vi "AutonomousVelocity.vi"() -> (0 "Terminate":bool)   [LabVIEW 2015]
uses:
  <vilib>/Rock Robotics/WPI/DriverStation/WPI_DriverStationRobotMode2.ctl
  <vilib>/Rock Robotics/WPI/CAN/TalonSRX/WPI_CANTalonSRX_APIControlMode.ctl
  <vilib>/Rock Robotics/WPI/Solenoid/WPI_SolenoidValue.ctl
  Utilities/AutoVars.vi
  Utilities/MotorPositionGlobals.vi
  Utilities/ShiftGlobals.vi
  Utilities/GlobalVisionVars.vi
  Utilities/VisionGlobals.vi
  <vilib>/Rock Robotics/WPI/Solenoid/WPI_SolenoidSetEnum.vi
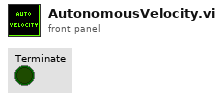
[diagram p1: front panel]
types:
  T1 = enum16{"WaitingForInput", "Driving", "TurnToTarget", "DriveMore", "Shoot", "End"}
  T2 = typedef "WPI_DriverStationRobotMode2.ctl" = enum16{"Autonomous Disabled", "Autonomous Enabled", "Teleop Disabled", "Teleop Enabled", "Disconnected", "Finish", "Test Disabled", "Test Enabled", "Emergency Stopped"}
  T3 = enum16{"Far Left", "Pos 2", "Pos 3", "Pos 4", "Far Right"}
  T4 = typedef "WPI_SolenoidValue.ctl" = enum16{"Off", "On", "Forward", "Reverse"}
  T5 = typedef "WPI_MotorControlDeviceRef.ctl" = cluster{"DeviceStatus":errorcluster, "Type":T6, "PWM":cluster{"PWM Channel":T7, "DeadBand":T8}, "CAN":cluster{"Device Number":u8, "Control Mode":T9, "Semaphore":T10, "Max Vout":dbl, "TalonSRX Control Mode":T11}, "Invert":bool}
  T6 = typedef "WPI_MotorControlType.ctl" = enum16{"PWM", "CAN", "CANTalonSRX"}
  T7 = typedef "FPGA_DIOPWMChannel.ctl" = enum8{"PWM 0", "PWM 1", "PWM 2", "PWM 3", "PWM 4", "PWM 5", "PWM 6", "PWM 7", "PWM 8", "PWM 9", "PWM MXP 0", "PWM MXP 1", "PWM MXP 2", "PWM MXP 3", "PWM MXP 4", "PWM MXP 5", "PWM MXP 6", "PWM MXP 7", "PWM MXP 8", "PWM MXP 9", "Invalid"}
  T8 = typedef "WPI_PWMDeadband.ctl" = cluster{"Name":string, "maxPositivePwm":i32, "minPositivePwm":i32, "centerPwm":i32, "maxNegativePwm":i32, "minNegativePwm":i32, "angularRange":u16}
  T9 = typedef "WPI_CANJaguar_ControlMode.ctl" = enum8{"Percent VBus", "Current", "Speed", "Position", "Voltage"}
  T10 = typedef "Semaphore RefNum" = refnum<k1>
  T11 = typedef "WPI_CANTalonSRX_APIControlMode.ctl" = enum8{"Percent VBus", "Speed", "Position", "Slave", "Unchanged / Invalid", "Voltage Compensation", "Current", "Motion Profile"}
  T12 = typedef "WPI_CANTalonSRX_GlobalStatus.ctl" = cluster{"Applied Throttle":dbl, "Module Enabled":bool, "CAN Error":errorcluster, "Closed Loop Error":dbl, "Forward Limit Switch Closed":bool, "Reverse Limit Switch Closed":bool, "Sensor Position":dbl, "Sensor Velocity":dbl, "Current":dbl, "Sticky Fault - Over Temp":bool, "Sticky Fault - Under Voltage":bool, "Sticky Fault - Forward Limit":bool, "Sticky Fault - Reverse Limit":bool, "Sticky Fault - Forward Soft Limit":bool, "Sticky Fault - Reverse Soft Limit":bool, "Brake is Enabled":bool, "Encoder Position":dbl, "Encoder Velocity":dbl, "Encoder Index Count":dbl, "Encoder A Pin State":bool, "Encoder B Pin State":bool, "Encoder Index Pin State":bool, "Analog In":dbl, "Analog In Velocity":dbl, "Temperature (C)":dbl, "Battery Voltage":dbl, "Control 5 Is Supported":bool, "Current Profile Slot Select":dbl, "Pos Div 8":bool, "Vel Div 4":bool, "Pulse Width Position":i32, "Pulse Width Velocity":i32, "Pulse Width Rise To Rise (us)":i32, "Pulse Width Rise To Fall (us)":i32, "Mot Prof Active Is Under Run":bool, "Mot Prof Active Has Under Run":bool, "Mot Prof Active Is Last":bool, "Mot Prof Active Velocity Only":bool, "Mot Prof Active Is Valid":bool, "Mot Prof Buffer Is Full":bool, "Mot Prof Active Profile Slot Select":i32, "Mot Prof NextID":i32, "Mot Prof Count":i32, "Mot Prof Active Velocity":dbl, "Mot Prof Active Position":dbl, "Mot Prof Output Enable":i32}
  T13 = typedef "WPI_DigitalOutputDevRef.ctl" = cluster{"DIO Channel":T14, "DevStatus":errorcluster}
  T14 = typedef "FPGA_DIOChannel.ctl" = enum8{"DIO 0", "DIO 1", "DIO 2", "DIO 3", "DIO 4", "DIO 5", "DIO 6", "DIO 7", "DIO 8", "DIO 9", "DIO MXP 0", "DIO MXP 1", "DIO MXP 2", "DIO MXP 3", "DIO MXP 4", "DIO MXP 5", "DIO MXP 6", "DIO MXP 7", "DIO MXP 8", "DIO MXP 9", "DIO MXP 10", "DIO MXP 11", "DIO MXP 12", "DIO MXP 13", "DIO MXP 14", "DIO MXP 15", "Invalid"}
  T15 = typedef "WPI_GyroDevRef.ctl" = cluster{"DevStatus":errorcluster, "Analog Channel":T16, "Offset":dbl, "Gain (VoltsPerDegree/Second)":dbl, "Gyro Type":enum16{"Analog", "XRS450"}, "Handle":i32, "SPI Bus":T17, "Device Found":bool, "Sample Rate":dbl, "Calibrate On Open":bool}
  T16 = typedef "FPGA_AIChannel.ctl" = enum8{"AI 0", "AI 1", "AI 2", "AI 3", "AI MXP 0", "AI MXP 1", "AI MXP 2", "AI MXP 3", "Invalid"}
  T17 = typedef "spi_bus.ctl" = enum16{"SPI On-Board, CS0", "SPI On-Board, CS1", "SPI On-Board, CS2", "SPI On-Board, CS3", "SPI MXP", "Invalid"}
  T18 = typedef "WPI_SolenoidDevRef.ctl" = cluster{"DevStatus":errorcluster, "Pneumatics Control Module":u8, "Forward Solenoid Channel":T19, "Reverse Solenoid Channel":T19}
  T19 = typedef "WPI_SolenoidChannel.ctl" = enum8{"Solenoid 0", "Solenoid 1", "Solenoid 2", "Solenoid 3", "Solenoid 4", "Solenoid 5", "Solenoid 6", "Solenoid 7", "Invalid"}
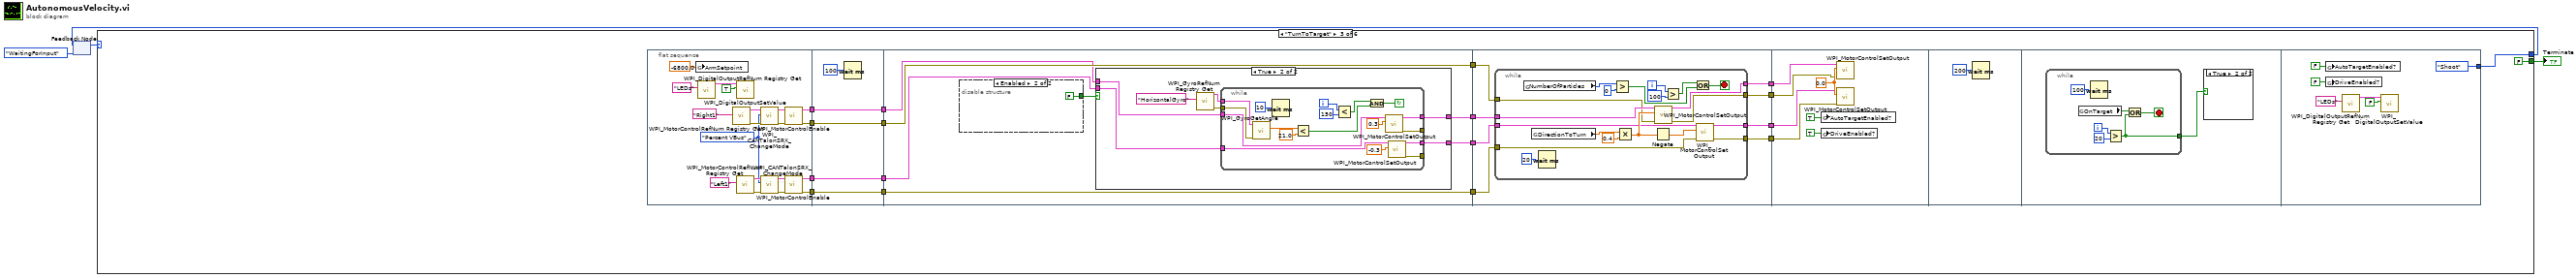
[diagram p0: block diagram]
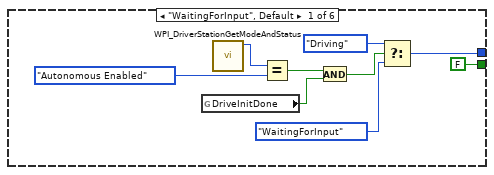
[diagram p2: hidden frame]
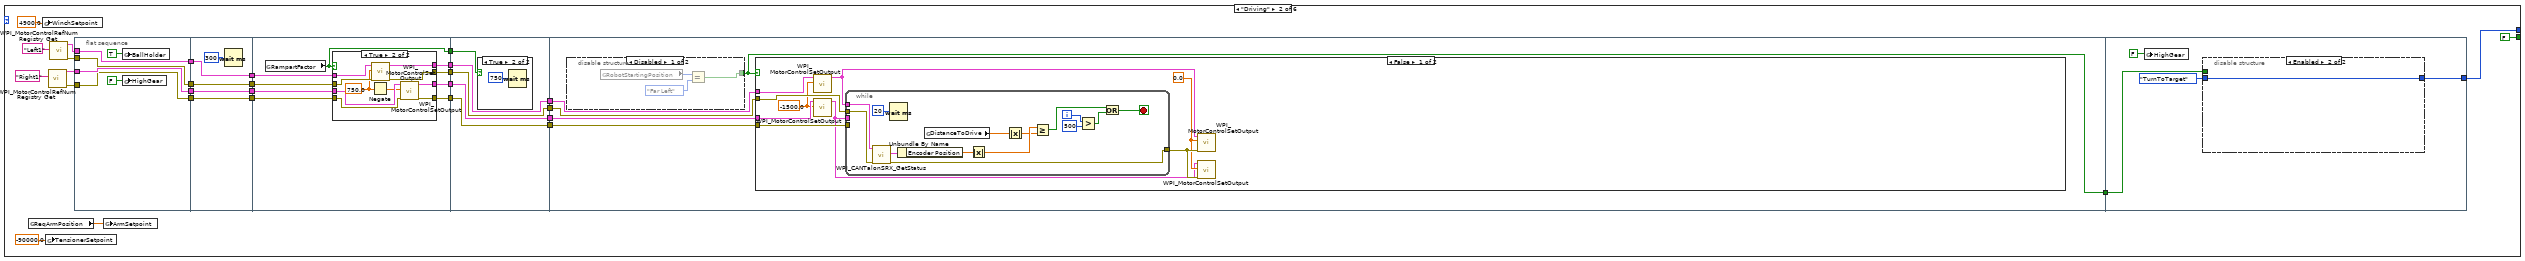
[diagram p3: hidden frame]
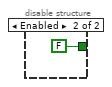
[diagram p6: hidden frame]
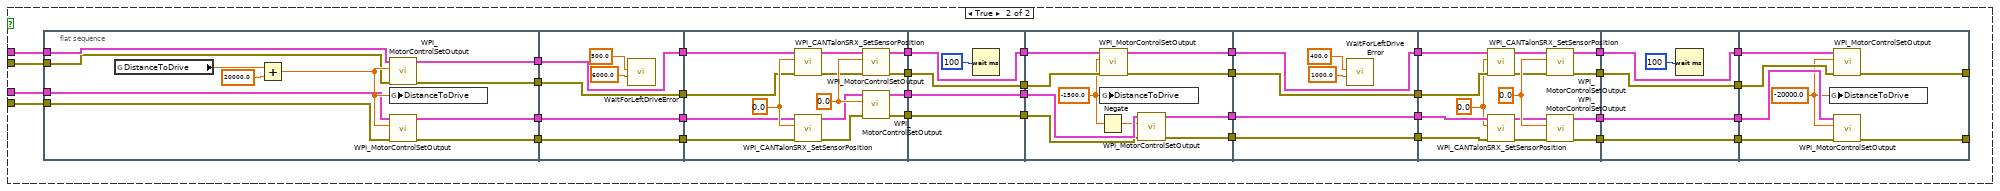
[diagram p7: hidden frame]
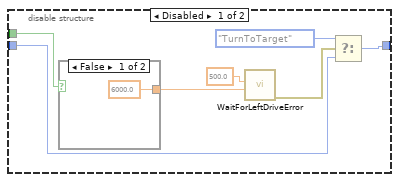
[diagram p8: hidden frame]
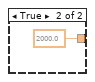
[diagram p9: hidden frame]
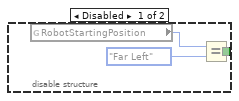
[diagram p10: hidden frame]
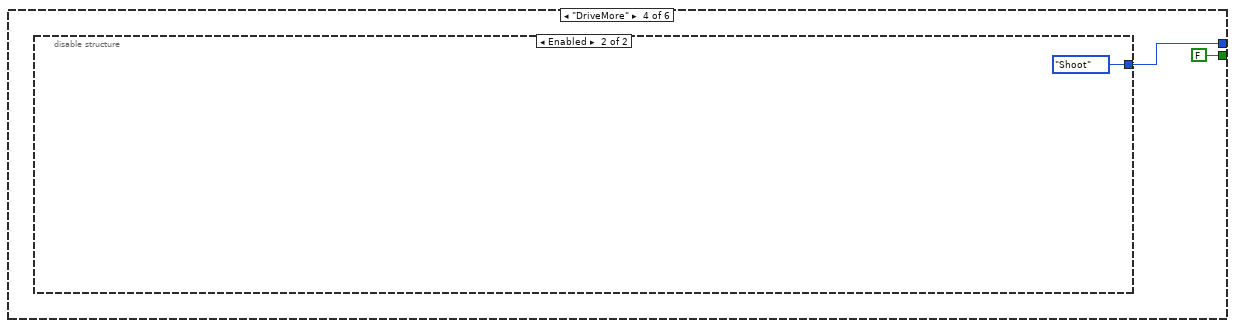
[diagram p13: hidden frame]
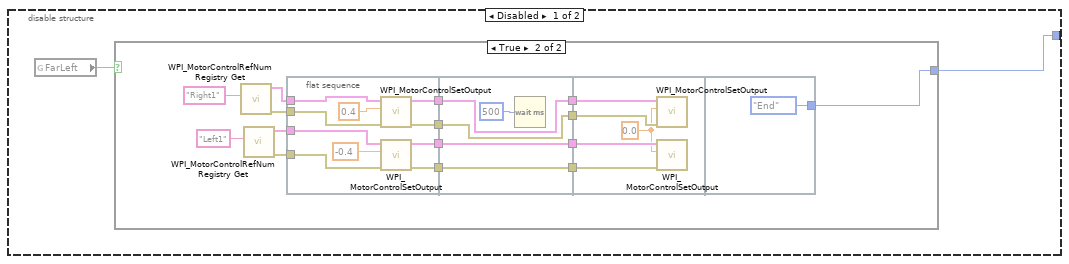
[diagram p14: hidden frame]
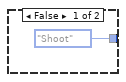
[diagram p15: hidden frame]
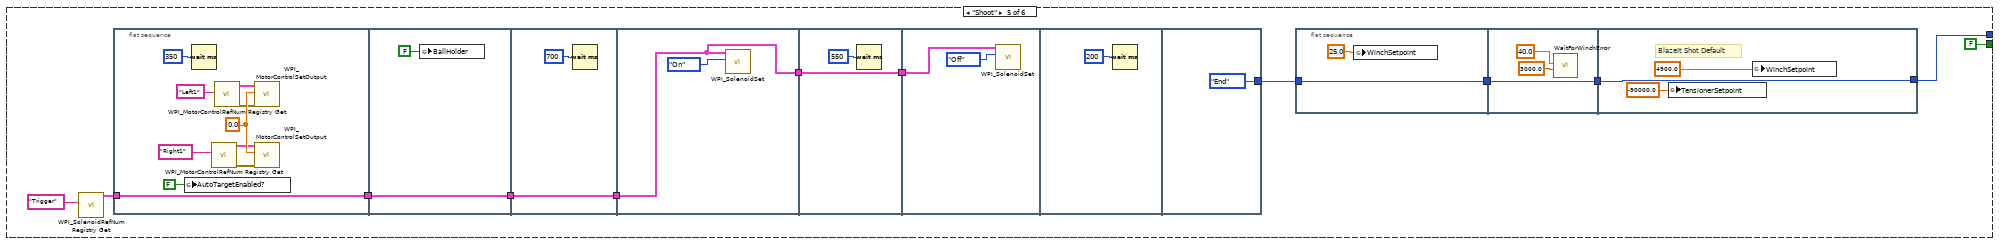
[diagram p16: hidden frame]
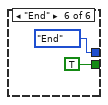
[diagram p17: hidden frame]
diagram:
  n1 = feedback #1(T1."WaitingForInput" ("AutoStateMachine")) -> (w1:T1)
  n2 = case shown="\"TurnToTarget\"" w1 {
    tunnel: [w13 w25 w260 w373 w416 T1."End" ("AutoStateMachine")] -> w4
    tunnel: [FALSE FALSE FALSE FALSE FALSE TRUE] -> w3
    frame "WaitingForInput", Default {
      n3 = global read "AutoVars.vi" "DriveInitDone"() -> (w8:bool)
      n4 = call <vilib>:"WPI_DriverStationGetModeAndStatus.vi"() -> ("Robot Mode"=w11:T2)  [unwired: 10 in, 1 out]
      n5 = Equal?(x=w11, y=WPI_DriverStationRobotMode2."Autonomous Enabled" ("Robot Mode")) -> (x = y?=w9:bool)
      n6 = And(x=w9, y=w8) -> (x .and. y?=w7:bool)
      n7 = Select(t=T1."Driving" ("AutoStateMachine"), s=w7, f=T1."WaitingForInput" ("AutoStateMachine")) -> (s? t:f=w13:T1)
    }
    frame "Driving" {
      n8 = global read "AutoVars.vi" "ReqArmPosition"() -> (w24:dbl)
      n9 = global write "MotorPositionGlobals.vi" "WinchSetpoint"(4900.0 ("WinchSetpoint")) -> ()
      n10 = global write "MotorPositionGlobals.vi" "TensionerSetpoint"(-90000.0 ("TensionerSetpoint")) -> ()
      n11 = call <vilib>:"WPI_MotorControlRefNum Registry Get.vi"("refnum name"="Right1") -> ("error out"=w36:errorcluster, "MotorControlDevRef"=w37:T5)  [unwired: 9 in]
      n12 = call <vilib>:"WPI_MotorControlRefNum Registry Get.vi"("refnum name"="Left1") -> ("error out"=w34:errorcluster, "MotorControlDevRef"=w35:T5)  [unwired: 9 in]
      n13 = flat-sequence {
        tunnel: w34 -> [w45]
        tunnel: w35 -> [w46]
        tunnel: w36 -> [w47]
        tunnel: w37 -> [w48]
        tunnel: [w48] -> w23
        tunnel: [w47] -> w21
        tunnel: [w46] -> w19
        tunnel: [w45] -> w17
        tunnel: w23 -> [w53]
        tunnel: [w53] -> w22
        tunnel: w21 -> [w52]
        tunnel: [w52] -> w20
        tunnel: w19 -> [w51]
        tunnel: [w51] -> w18
        tunnel: w17 -> [w50]
        tunnel: [w50] -> w16
        tunnel: [w58] -> w33
        tunnel: [w57] -> w31
        tunnel: [w56] -> w29
        tunnel: [w55] -> w27
        tunnel: w22 -> [w62]
        tunnel: w20 -> [w61]
        tunnel: w18 -> [w60]
        tunnel: w16 -> [w59]
        tunnel: [w54] -> w15
        tunnel: w33 -> [w81]
        tunnel: [w81] -> w32
        tunnel: w31 -> [w80]
        tunnel: [w80] -> w30
        tunnel: w29 -> [w79]
        tunnel: [w79] -> w28
        tunnel: w27 -> [w78]
        tunnel: [w78] -> w26
        tunnel: w15 -> [w77]
        tunnel: w32 -> [w87]
        tunnel: w30 -> [w86]
        tunnel: w28 -> [w84]
        tunnel: w26 -> [w85]
        tunnel: [w83] -> w14
        tunnel: [w231] -> w25
        tunnel: w14 -> [w230]
        frame #0 {
          n14 = global write "MotorPositionGlobals.vi" "BallHolder"(TRUE ("BallHolder")) -> ()
          n15 = global write "ShiftGlobals.vi" "HighGear"(FALSE ("HighGear")) -> ()
        }
        frame #1 {
          n16 = Wait (ms)(milliseconds to wait=u32 300) -> ()  [unwired: 1 out]
        }
        frame #2 {
          n17 = global read "AutoVars.vi" "RampartFactor"() -> (w54:bool)
          n18 = case shown="True" w54 {
            tunnel: w62 -> [w64 w76]
            tunnel: w61 -> [w63 w75]
            tunnel: w60 -> [w66 w74]
            tunnel: w59 -> [w65 w73]
            tunnel: [w64 w72] -> w58
            tunnel: [w63 w71] -> w57
            tunnel: [w66 w70] -> w56
            tunnel: [w65 w69] -> w55
            frame False {
            }
            frame True {
              w68 = 750.0
              n19 = Negate(x=w68) -> (-x=w67:dbl)
              n20 = call <vilib>:"WPI_MotorControlSetOutput.vi"("error in (no error)"=w73, "Output"=w68, "MotorControlDevRef"=w74) -> ("error out"=w69:errorcluster, "MotorControlDevRef"=w70:T5)  [unwired: 6 in, 1 out]
              n21 = call <vilib>:"WPI_MotorControlSetOutput.vi"("error in (no error)"=w75, "Output"=w67, "MotorControlDevRef"=w76) -> ("error out"=w71:errorcluster, "MotorControlDevRef"=w72:T5)  [unwired: 6 in, 1 out]
            }
          }
        }
        frame #3 {
          n22 = case shown="True" w77 {
            frame False {
            }
            frame True {
              n23 = Wait (ms)(milliseconds to wait=u32 750) -> ()  [unwired: 1 out]
            }
          }
        }
        frame #4 {
          n24 = disable-structure shown="Disabled" {
            disable-tunnel: [w88 FALSE] -> w83
            frame Disabled {
              n25 = global read "AutoVars.vi" "RobotStartingPosition"() -> (w90:T3)
              n26 = Equal?(x=w90, y=T3."Far Left") -> (x = y?=w88:bool)
            }
            frame Enabled {
            }
          }
          n27 = case shown="False" w83 {
            tunnel: w87 -> [w94 w149]
            tunnel: w86 -> [w99 w147]
            tunnel: w85 -> [w100 w148]
            tunnel: w84 -> [w96 w150]
            frame False {
              w92 = -1500.0 ("Output")
              w97 = 0.0 ("Output")
              n28 = call <vilib>:"WPI_MotorControlSetOutput.vi"("Output"=w92, "MotorControlDevRef"=w96) -> ("MotorControlDevRef"=w95:T5)  [unwired: 7 in, 2 out]
              n29 = call <vilib>:"WPI_MotorControlSetOutput.vi"("Output"=w92, "MotorControlDevRef"=w94) -> ("MotorControlDevRef"=w93:T5)  [unwired: 7 in, 2 out]
              n30 = while {
                tunnel: w93 -> [_]
                tunnel: w95 -> [w102]
                tunnel: w100 -> [w101]
                tunnel: w99 -> [_]
                tunnel: [w111] -> w98
                i -> [w107]
                stop <- w109 stop-if-true
                n31 = call <vilib>:"WPI_CANTalonSRX_GetStatus.vi"("error in (no error)"=w101, "CAN Talon SRX Ref"=w102) -> ("error out"=w111:errorcluster, "Talon SRX Status"=w113:T12)  [unwired: 7 in, 1 out]
                n32 = Wait (ms)(milliseconds to wait=u32 20) -> ()  [unwired: 1 out]
                n33 = Unbundle By Name(w113) -> ("Encoder Position"=w105:dbl)
                n34 = global read "AutoVars.vi" "DistanceToDrive"() -> (w112:dbl)
                n35 = Absolute Value(x=w105) -> (abs(x)=w104:dbl)
                n36 = Absolute Value(x=w112) -> (abs(x)=w103:dbl)
                n37 = Greater Or Equal?(x=w104, y=w103) -> (x >= y?=w110:bool)
                n38 = Greater?(x=w107, y=500) -> (0:w108:bool)
                n39 = Or(x=w110, y=w108) -> (x .or. y?=w109:bool)
              }
              n40 = call <vilib>:"WPI_MotorControlSetOutput.vi"("error in (no error)"=w98, "Output"=w97, "MotorControlDevRef"=w95) -> ()  [unwired: 6 in, 3 out]
              n41 = call <vilib>:"WPI_MotorControlSetOutput.vi"("error in (no error)"=w98, "Output"=w97, "MotorControlDevRef"=w93) -> ()  [unwired: 6 in, 3 out]
            }
            frame True {
              n42 = flat-sequence {
                tunnel: w150 -> [w158]
                tunnel: w149 -> [w157]
                tunnel: w148 -> [w156]
                tunnel: w147 -> [w155]
                tunnel: [w154] -> w145
                tunnel: [w153] -> w143
                tunnel: [w152] -> w141
                tunnel: [w151] -> w140
                tunnel: [w165] -> w146
                tunnel: w145 -> [w165]
                tunnel: [w164] -> w144
                tunnel: w143 -> [w164]
                tunnel: [w163] -> w142
                tunnel: w141 -> [w163]
                tunnel: w140 -> [w162]
                tunnel: [w162] -> w139
                tunnel: w146 -> [w175]
                tunnel: w144 -> [w174]
                tunnel: w142 -> [w173]
                tunnel: w139 -> [w172]
                tunnel: [w171] -> w130
                tunnel: [w170] -> w128
                tunnel: [w169] -> w126
                tunnel: [w168] -> w124
                tunnel: w130 -> [w186]
                tunnel: [w186] -> w129
                tunnel: w128 -> [w185]
                tunnel: [w185] -> w127
                tunnel: w126 -> [w184]
                tunnel: [w184] -> w125
                tunnel: w124 -> [w183]
                tunnel: [w183] -> w123
                tunnel: w129 -> [w196]
                tunnel: w127 -> [w195]
                tunnel: w125 -> [w194]
                tunnel: w123 -> [w193]
                tunnel: [w192] -> w138
                tunnel: [w191] -> w136
                tunnel: [w190] -> w134
                tunnel: [w189] -> w132
                tunnel: w138 -> [w202]
                tunnel: [w202] -> w137
                tunnel: w136 -> [w201]
                tunnel: [w201] -> w135
                tunnel: w134 -> [w200]
                tunnel: [w200] -> w133
                tunnel: w132 -> [w199]
                tunnel: [w199] -> w131
                tunnel: w137 -> [w215]
                tunnel: w135 -> [w214]
                tunnel: w133 -> [w213]
                tunnel: w131 -> [w212]
                tunnel: [w210] -> w116
                tunnel: [w209] -> w118
                tunnel: [w208] -> w120
                tunnel: [w207] -> w122
                tunnel: w122 -> [w221]
                tunnel: [w221] -> w121
                tunnel: w120 -> [w220]
                tunnel: [w220] -> w119
                tunnel: w118 -> [w219]
                tunnel: [w219] -> w117
                tunnel: w116 -> [w218]
                tunnel: [w218] -> w115
                tunnel: w121 -> [w225]
                tunnel: w119 -> [w226]
                tunnel: w117 -> [w227]
                tunnel: w115 -> [w228]
                tunnel: [w224] -> _
                tunnel: [w223] -> _
                frame #0 {
                  n43 = global read "AutoVars.vi" "DistanceToDrive"() -> (w160:dbl)
                  n44 = Add(x=w160, y=20000.0) -> (x+y=w159:dbl)
                  n45 = call <vilib>:"WPI_MotorControlSetOutput.vi"("error in (no error)"=w156, "Output"=w159, "MotorControlDevRef"=w158) -> ("error out"=w153:errorcluster, "MotorControlDevRef"=w154:T5)  [unwired: 6 in, 1 out]
                  n46 = global write "AutoVars.vi" "DistanceToDrive"(w159) -> ()
                  n47 = call <vilib>:"WPI_MotorControlSetOutput.vi"("error in (no error)"=w155, "Output"=w159, "MotorControlDevRef"=w157) -> ("error out"=w151:errorcluster, "MotorControlDevRef"=w152:T5)  [unwired: 6 in, 1 out]
                }
                frame #1 {
                  n48 = call "WaitForLeftDriveError.vi"("Timeout (ms)"=6000.0, "AllowedError"=500.0) -> ()  [unwired: 9 in, 1 out]
                }
                frame #2 {
                  w180 = 0.0 ("New Sensor Position")
                  w181 = 0.0 ("Output")
                  n49 = call <vilib>:"WPI_CANTalonSRX_SetSensorPosition.vi"("error in (no error)"=w174, "New Sensor Position"=w180, "CAN Talon SRX Ref"=w175) -> ("error out"=w178:errorcluster, "CAN Talon SRX Ref"=w179:T5)  [unwired: 7 in]
                  n50 = call <vilib>:"WPI_CANTalonSRX_SetSensorPosition.vi"("error in (no error)"=w172, "New Sensor Position"=w180, "CAN Talon SRX Ref"=w173) -> ("error out"=w176:errorcluster, "CAN Talon SRX Ref"=w177:T5)  [unwired: 7 in]
                  n51 = call <vilib>:"WPI_MotorControlSetOutput.vi"("error in (no error)"=w178, "Output"=w181, "MotorControlDevRef"=w179) -> ("error out"=w170:errorcluster, "MotorControlDevRef"=w171:T5)  [unwired: 6 in, 1 out]
                  n52 = call <vilib>:"WPI_MotorControlSetOutput.vi"("error in (no error)"=w176, "Output"=w181, "MotorControlDevRef"=w177) -> ("error out"=w168:errorcluster, "MotorControlDevRef"=w169:T5)  [unwired: 6 in, 1 out]
                }
                frame #3 {
                  n53 = Wait (ms)(milliseconds to wait=u32 100) -> ()  [unwired: 1 out]
                }
                frame #4 {
                  w187 = -1500.0
                  n54 = Negate(x=w187) -> (-x=w188:dbl)
                  n55 = call <vilib>:"WPI_MotorControlSetOutput.vi"("error in (no error)"=w195, "Output"=w187, "MotorControlDevRef"=w196) -> ("error out"=w191:errorcluster, "MotorControlDevRef"=w192:T5)  [unwired: 6 in, 1 out]
                  n56 = global write "AutoVars.vi" "DistanceToDrive"(w187) -> ()
                  n57 = call <vilib>:"WPI_MotorControlSetOutput.vi"("error in (no error)"=w193, "Output"=w188, "MotorControlDevRef"=w194) -> ("error out"=w189:errorcluster, "MotorControlDevRef"=w190:T5)  [unwired: 6 in, 1 out]
                }
                frame #5 {
                  n58 = call "WaitForLeftDriveError.vi"("Timeout (ms)"=1000.0, "AllowedError"=400.0) -> ()  [unwired: 9 in, 1 out]
                }
                frame #6 {
                  w211 = 0.0 ("New Sensor Position")
                  w216 = 0.0 ("Output")
                  n59 = call <vilib>:"WPI_CANTalonSRX_SetSensorPosition.vi"("error in (no error)"=w214, "New Sensor Position"=w211, "CAN Talon SRX Ref"=w215) -> ("error out"=w205:errorcluster, "CAN Talon SRX Ref"=w206:T5)  [unwired: 7 in]
                  n60 = call <vilib>:"WPI_CANTalonSRX_SetSensorPosition.vi"("error in (no error)"=w212, "New Sensor Position"=w211, "CAN Talon SRX Ref"=w213) -> ("error out"=w203:errorcluster, "CAN Talon SRX Ref"=w204:T5)  [unwired: 7 in]
                  n61 = call <vilib>:"WPI_MotorControlSetOutput.vi"("error in (no error)"=w205, "Output"=w216, "MotorControlDevRef"=w206) -> ("error out"=w209:errorcluster, "MotorControlDevRef"=w210:T5)  [unwired: 6 in, 1 out]
                  n62 = call <vilib>:"WPI_MotorControlSetOutput.vi"("error in (no error)"=w203, "Output"=w216, "MotorControlDevRef"=w204) -> ("error out"=w207:errorcluster, "MotorControlDevRef"=w208:T5)  [unwired: 6 in, 1 out]
                }
                frame #7 {
                  n63 = Wait (ms)(milliseconds to wait=u32 100) -> ()  [unwired: 1 out]
                }
                frame #8 {
                  w222 = -20000.0 ("Output")
                  n64 = global write "AutoVars.vi" "DistanceToDrive"(w222) -> ()
                  n65 = call <vilib>:"WPI_MotorControlSetOutput.vi"("error in (no error)"=w227, "Output"=w222, "MotorControlDevRef"=w228) -> ("error out"=w224:errorcluster)  [unwired: 6 in, 2 out]
                  n66 = call <vilib>:"WPI_MotorControlSetOutput.vi"("error in (no error)"=w225, "Output"=w222, "MotorControlDevRef"=w226) -> ("error out"=w223:errorcluster)  [unwired: 6 in, 2 out]
                }
              }
            }
          }
        }
        frame #5 {
          n67 = global write "ShiftGlobals.vi" "HighGear"(FALSE ("HighGear")) -> ()
          n68 = disable-structure shown="Enabled" {
            disable-tunnel: T1."TurnToTarget" ("AutoStateMachine") -> [w236 w242]
            disable-tunnel: [w234 w242] -> w231
            disable-tunnel: w230 -> [w233 _]
            frame Disabled {
              n69 = case shown="False" w233 {
                tunnel: [6000.0 ("Timeout (ms)") 2000.0 ("Timeout (ms)")] -> w239
                frame False {
                }
                frame True {
                }
              }
              n70 = call "WaitForLeftDriveError.vi"("Timeout (ms)"=w239, "AllowedError"=500.0) -> ("error out"=w237:errorcluster)  [unwired: 9 in]
              n71 = Select(t=T1."TurnToTarget", s=w237, f=w236) -> (s? t:f=w234:T1)
            }
            frame Enabled {
            }
          }
        }
      }
      n72 = global write "MotorPositionGlobals.vi" "ArmSetpoint"(w24) -> ()
    }
    frame "TurnToTarget" {
      n73 = flat-sequence {
        tunnel: [w268] -> w258
        tunnel: [w267] -> w257
        tunnel: [w266] -> w256
        tunnel: [w265] -> w255
        tunnel: w258 -> [w281]
        tunnel: w257 -> [w280]
        tunnel: w256 -> [w283]
        tunnel: w255 -> [w282]
        tunnel: [w283] -> w250
        tunnel: [w282] -> w248
        tunnel: [w281] -> w246
        tunnel: [w280] -> w244
        tunnel: w250 -> [w288]
        tunnel: [w287] -> w249
        tunnel: w248 -> [w291]
        tunnel: [w291] -> w247
        tunnel: w246 -> [w286]
        tunnel: [w285] -> w245
        tunnel: w244 -> [w290]
        tunnel: [w290] -> w243
        tunnel: [w330] -> w254
        tunnel: [w329] -> w253
        tunnel: [w328] -> w252
        tunnel: [w327] -> w251
        tunnel: w249 -> [w326]
        tunnel: w247 -> [w325]
        tunnel: w245 -> [w324]
        tunnel: w243 -> [w323]
        tunnel: w254 -> [w354]
        tunnel: w253 -> [w353]
        tunnel: w252 -> [w352]
        tunnel: w251 -> [w351]
        tunnel: [T1."Shoot" ("AutoStateMachine")] -> w260
        frame #0 {
          w273 = WPI_CANTalonSRX_APIControlMode."Percent VBus" ("Control Mode")
          n74 = global write "MotorPositionGlobals.vi" "ArmSetpoint"(-6800.0 ("ArmSetpoint")) -> ()
          n75 = call <vilib>:"WPI_DigitalOutputRefNum Registry Get.vi"("refnum name"="LEDs") -> ("DigitalOutputDevRef"=w263:T13)  [unwired: 9 in, 1 out]
          n76 = call <vilib>:"WPI_MotorControlRefNum Registry Get.vi"("refnum name"="Right1") -> ("error out"=w277:errorcluster, "MotorControlDevRef"=w276:T5)  [unwired: 9 in]
          n77 = call <vilib>:"WPI_MotorControlRefNum Registry Get.vi"("refnum name"="Left1") -> ("error out"=w275:errorcluster, "MotorControlDevRef"=w274:T5)  [unwired: 9 in]
          n78 = call <vilib>:"WPI_DigitalOutputSetValue.vi"("Value"=TRUE, "DigitalOutputDevRef"=w263) -> ()  [unwired: 8 in, 2 out]
          n79 = call <vilib>:"WPI_CANTalonSRX_ChangeMode.vi"("error in (no error)"=w277, "Control Mode"=w273, "CAN Talon SRX Ref"=w276) -> ("error out"=w271:errorcluster, "CAN Talon SRX Ref"=w272:T5)  [unwired: 7 in]
          n80 = call <vilib>:"WPI_CANTalonSRX_ChangeMode.vi"("error in (no error)"=w275, "Control Mode"=w273, "CAN Talon SRX Ref"=w274) -> ("error out"=w269:errorcluster, "CAN Talon SRX Ref"=w270:T5)  [unwired: 7 in]
          n81 = call <vilib>:"WPI_MotorControlEnable.vi"("error in (no error)"=w271, "CAN MotorDevRef"=w272) -> ("error out"=w265:errorcluster, "CAN MotorDevRef"=w266:T5)  [unwired: 8 in]
          n82 = call <vilib>:"WPI_MotorControlEnable.vi"("error in (no error)"=w269, "CAN MotorDevRef"=w270) -> ("error out"=w267:errorcluster, "CAN MotorDevRef"=w268:T5)  [unwired: 8 in]
        }
        frame #1 {
          n83 = Wait (ms)(milliseconds to wait=u32 100) -> ()  [unwired: 1 out]
        }
        frame #2 {
          n84 = disable-structure shown="Enabled" {
            disable-tunnel: [w292 FALSE] -> w289
            frame Disabled {
              n85 = global read "AutoVars.vi" "RobotStartingPosition"() -> (w294:T3)
              n86 = Equal?(x=w294, y=T3."Far Left") -> (x = y?=w292:bool)
            }
            frame Enabled {
            }
          }
          n87 = case shown="True" w289 {
            tunnel: w288 -> [w297 w304]
            tunnel: [w297 w303] -> w287
            tunnel: w286 -> [w296 w302]
            tunnel: [w296 w301] -> w285
            frame False {
            }
            frame True {
              n88 = call <vilib>:"WPI_GyroRefNum Registry Get.vi"("refnum name"="HorizontalGyro") -> ("error out"=w298:errorcluster, "GyroDevRef"=w299:T15)  [unwired: 9 in]
              n89 = while {
                tunnel: w302 -> [w320]
                tunnel: w304 -> [w319]
                tunnel: [w318] -> w301
                tunnel: [w317] -> _
                tunnel: [w316] -> w303
                tunnel: [w315] -> _
                tunnel: w299 -> [w314]
                tunnel: w298 -> [w313]
                i -> [w306]
                stop <- w309 continue-if-true
                n90 = call <vilib>:"WPI_GyroGetAngle.vi"("error in"=w313, "GyroDevRef"=w314) -> ("Angle"=w312:dbl)  [unwired: 5 in, 4 out]
                n91 = Wait (ms)(milliseconds to wait=u32 10) -> ()  [unwired: 1 out]
                n92 = Less?(x=w312, y=21.0) -> (x < y?=w308:bool)
                n93 = Less?(x=w306, y=150) -> (x < y?=w307:bool)
                n94 = And(x=w307, y=w308) -> (x .and. y?=w309:bool)
                n95 = call <vilib>:"WPI_MotorControlSetOutput.vi"("Output"=0.3, "MotorControlDevRef"=w319) -> ("error out"=w315:errorcluster, "MotorControlDevRef"=w316:T5)  [unwired: 7 in, 1 out]
                n96 = call <vilib>:"WPI_MotorControlSetOutput.vi"("Output"=-0.3, "MotorControlDevRef"=w320) -> ("error out"=w317:errorcluster, "MotorControlDevRef"=w318:T5)  [unwired: 7 in, 1 out]
              }
            }
          }
        }
        frame #3 {
          n97 = while {
            tunnel: [w343] -> w330
            tunnel: [w342] -> w329
            tunnel: [w341] -> w328
            tunnel: [w340] -> w327
            tunnel: w326 -> [w339]
            tunnel: w325 -> [w338]
            tunnel: w324 -> [w337]
            tunnel: w323 -> [w336]
            i -> [w332]
            stop <- w335 stop-if-true
            n98 = global read "GlobalVisionVars.vi" "NumberOfParticles"() -> (w350:i32)
            n99 = global read "AutoVars.vi" "DirectionToTurn"() -> (w347:dbl)
            n100 = Wait (ms)(milliseconds to wait=u32 20) -> ()  [unwired: 1 out]
            n101 = Greater?(x=w350, y=0) -> (0:w334:bool)
            n102 = Multiply(x=w347, y=0.4) -> (x*y=w344:dbl)
            n103 = Negate(x=w344) -> (-x=w345:dbl)
            n104 = call <vilib>:"WPI_MotorControlSetOutput.vi"("error in (no error)"=w338, "Output"=w344, "MotorControlDevRef"=w339) -> ("error out"=w342:errorcluster, "MotorControlDevRef"=w343:T5)  [unwired: 6 in, 1 out]
            n105 = Greater?(x=w332, y=100) -> (0:w333:bool)
            n106 = Or(x=w333, y=w334) -> (x .or. y?=w335:bool)
            n107 = call <vilib>:"WPI_MotorControlSetOutput.vi"("error in (no error)"=w336, "Output"=w345, "MotorControlDevRef"=w337) -> ("error out"=w340:errorcluster, "MotorControlDevRef"=w341:T5)  [unwired: 6 in, 1 out]
          }
        }
        frame #4 {
          w356 = 0.0
          n108 = global write "VisionGlobals.vi" "AutoTargetEnabled?"(TRUE ("AutoTargetEnabled?")) -> ()
          n109 = global write "VisionGlobals.vi" "DriveEnabled?"(TRUE ("DriveEnabled?")) -> ()
          n110 = call <vilib>:"WPI_MotorControlSetOutput.vi"("error in (no error)"=w353, "Output"=w356, "MotorControlDevRef"=w354) -> ()  [unwired: 6 in, 3 out]
          n111 = call <vilib>:"WPI_MotorControlSetOutput.vi"("error in (no error)"=w351, "Output"=w356, "MotorControlDevRef"=w352) -> ()  [unwired: 6 in, 3 out]
        }
        frame #5 {
          n112 = Wait (ms)(milliseconds to wait=u32 200) -> ()  [unwired: 1 out]
        }
        frame #6 {
          n113 = while {
            tunnel: [w360] -> w359
            i -> [w362]
            stop <- w363 stop-if-true
            n114 = global read "GlobalVisionVars.vi" "OnTarget"() -> (w364:bool)
            n115 = Wait (ms)(milliseconds to wait=u32 100) -> ()  [unwired: 1 out]
            n116 = Greater?(x=w362, y=20) -> (0:w360:bool)
            n117 = Or(x=w364, y=w360) -> (x .or. y?=w363:bool)
          }
          n118 = case shown="True" w359 {
            frame False {
            }
            frame True {
            }
          }
        }
        frame #7 {
          n119 = global write "VisionGlobals.vi" "AutoTargetEnabled?"(FALSE ("AutoTargetEnabled?")) -> ()
          n120 = global write "VisionGlobals.vi" "DriveEnabled?"(FALSE ("DriveEnabled?")) -> ()
          n121 = call <vilib>:"WPI_DigitalOutputRefNum Registry Get.vi"("refnum name"="LEDs") -> ("DigitalOutputDevRef"=w369:T13)  [unwired: 9 in, 1 out]
          n122 = call <vilib>:"WPI_DigitalOutputSetValue.vi"("Value"=FALSE, "DigitalOutputDevRef"=w369) -> ()  [unwired: 8 in, 2 out]
        }
      }
    }
    frame "DriveMore" {
      n123 = disable-structure shown="Enabled" {
        disable-tunnel: [w375 T1."Shoot" ("AutoStateMachine")] -> w373
        frame Disabled {
          n124 = global read "AutoVars.vi" "FarLeft"() -> (w374:bool)
          n125 = case shown="True" w374 {
            tunnel: [T1."Shoot" ("AutoStateMachine") w389] -> w375
            frame False {
            }
            frame True {
              n126 = call <vilib>:"WPI_MotorControlRefNum Registry Get.vi"("refnum name"="Right1") -> ("error out"=w385:errorcluster, "MotorControlDevRef"=w386:T5)  [unwired: 9 in]
              n127 = call <vilib>:"WPI_MotorControlRefNum Registry Get.vi"("refnum name"="Left1") -> ("error out"=w387:errorcluster, "MotorControlDevRef"=w388:T5)  [unwired: 9 in]
              n128 = flat-sequence {
                tunnel: w388 -> [w401]
                tunnel: w387 -> [w400]
                tunnel: w386 -> [w399]
                tunnel: w385 -> [w398]
                tunnel: [w397] -> w384
                tunnel: [w396] -> w383
                tunnel: [w395] -> w382
                tunnel: [w394] -> w378
                tunnel: w384 -> [w404]
                tunnel: w383 -> [w402]
                tunnel: w382 -> [w405]
                tunnel: [w405] -> w381
                tunnel: [w404] -> w380
                tunnel: [w403] -> w379
                tunnel: w378 -> [w403]
                tunnel: [w402] -> w377
                tunnel: w381 -> [w411]
                tunnel: w380 -> [w410]
                tunnel: w379 -> [w409]
                tunnel: w377 -> [w408]
                tunnel: [T1."End" ("AutoStateMachine")] -> w389
                frame #0 {
                  n129 = call <vilib>:"WPI_MotorControlSetOutput.vi"("error in (no error)"=w398, "Output"=0.4, "MotorControlDevRef"=w399) -> ("error out"=w397:errorcluster, "MotorControlDevRef"=w395:T5)  [unwired: 6 in, 1 out]
                  n130 = call <vilib>:"WPI_MotorControlSetOutput.vi"("error in (no error)"=w400, "Output"=-0.4, "MotorControlDevRef"=w401) -> ("error out"=w396:errorcluster, "MotorControlDevRef"=w394:T5)  [unwired: 6 in, 1 out]
                }
                frame #1 {
                  n131 = Wait (ms)(milliseconds to wait=u32 500) -> ()  [unwired: 1 out]
                }
                frame #2 {
                  w407 = 0.0 ("Output")
                  n132 = call <vilib>:"WPI_MotorControlSetOutput.vi"("error in (no error)"=w410, "Output"=w407, "MotorControlDevRef"=w411) -> ()  [unwired: 6 in, 3 out]
                  n133 = call <vilib>:"WPI_MotorControlSetOutput.vi"("error in (no error)"=w408, "Output"=w407, "MotorControlDevRef"=w409) -> ()  [unwired: 6 in, 3 out]
                }
                frame #3 {
                }
              }
            }
          }
        }
        frame Enabled {
        }
      }
    }
    frame "Shoot" {
      n134 = call <vilib>:"WPI_SolenoidRefNum Registry Get.vi"("refnum name"="Trigger") -> ("SolenoidDevRef"=w421:T18)  [unwired: 9 in, 1 out]
      n135 = flat-sequence {
        tunnel: [w443] -> w415
        tunnel: w421 -> [w443]
        tunnel: w415 -> [w445]
        tunnel: [w445] -> w414
        tunnel: w414 -> [w447]
        tunnel: [w447] -> w425
        tunnel: [w448] -> w424
        tunnel: w425 -> [w448]
        tunnel: w424 -> [w450]
        tunnel: [w450] -> w423
        tunnel: w423 -> [w452]
        tunnel: [T1."End" ("AutoStateMachine")] -> w419
        frame #0 {
          w438 = 0.0
          n136 = global write "VisionGlobals.vi" "AutoTargetEnabled?"(FALSE ("AutoTargetEnabled?")) -> ()
          n137 = Wait (ms)(milliseconds to wait=u32 350) -> ()  [unwired: 1 out]
          n138 = call <vilib>:"WPI_MotorControlRefNum Registry Get.vi"("refnum name"="Right1") -> ("error out"=w436:errorcluster, "MotorControlDevRef"=w437:T5)  [unwired: 9 in]
          n139 = call <vilib>:"WPI_MotorControlRefNum Registry Get.vi"("refnum name"="Left1") -> ("error out"=w434:errorcluster, "MotorControlDevRef"=w435:T5)  [unwired: 9 in]
          n140 = call <vilib>:"WPI_MotorControlSetOutput.vi"("error in (no error)"=w434, "Output"=w438, "MotorControlDevRef"=w435) -> ()  [unwired: 6 in, 3 out]
          n141 = call <vilib>:"WPI_MotorControlSetOutput.vi"("error in (no error)"=w436, "Output"=w438, "MotorControlDevRef"=w437) -> ()  [unwired: 6 in, 3 out]
        }
        frame #1 {
          n142 = global write "MotorPositionGlobals.vi" "BallHolder"(FALSE ("BallHolder")) -> ()
        }
        frame #2 {
          n143 = Wait (ms)(milliseconds to wait=u32 700) -> ()  [unwired: 1 out]
        }
        frame #3 {
          n144 = call-poly <vilib>:"WPI_SolenoidSet.vi"("Value"=WPI_SolenoidValue."On", "SolenoidDevRef"=w448) -> ()  [unwired: 8 in, 2 out]
        }
        frame #4 {
          n145 = Wait (ms)(milliseconds to wait=u32 550) -> ()  [unwired: 1 out]
        }
        frame #5 {
          n146 = call-poly <vilib>:"WPI_SolenoidSet.vi"("Value"=WPI_SolenoidValue."Off", "SolenoidDevRef"=w452) -> ()  [unwired: 8 in, 2 out]
        }
        frame #6 {
          n147 = Wait (ms)(milliseconds to wait=u32 200) -> ()  [unwired: 1 out]
        }
        frame #7 {
        }
      }
      n148 = flat-sequence {
        tunnel: w419 -> [w426]
        tunnel: [w426] -> w417
        tunnel: [w428] -> w418
        tunnel: w417 -> [w428]
        tunnel: [w431] -> w416
        tunnel: w418 -> [w431]
        frame #0 {
          n149 = global write "MotorPositionGlobals.vi" "WinchSetpoint"(25.0 ("WinchPosition")) -> ()
        }
        frame #1 {
          n150 = call "WaitForWinchError.vi"("Timeout (ms)"=3000.0, "AllowedError"=40.0) -> ()  [unwired: 9 in, 1 out]
        }
        frame #2 {
          # "BlazeIt Shot Default"
          n151 = global write "MotorPositionGlobals.vi" "TensionerSetpoint"(-90000.0 ("TensionerSetpoint")) -> ()
          n152 = global write "MotorPositionGlobals.vi" "WinchSetpoint"(4900.0 ("WinchPosition")) -> ()
        }
      }
    }
    frame "End" {
    }
  }
  "Terminate" <- w3
  n153 = feedback-in #1(w4) -> ()
